vi "ReadSerialised String.vi"(8 "error in (no error)":errorcluster, 11 "object in":refnum<class "Message Class.lvclass">) -> (0 "error out":errorcluster, 2 "Serialised String":string, 3 "object out":refnum<class "Message Class.lvclass">)   [LabVIEW 2018, in "ClientMessaging.lvlib" / "Message Class.lvclass"]
uses:
  Message Class.lvclass
  Message Class.lvclass/Message Class.ctl
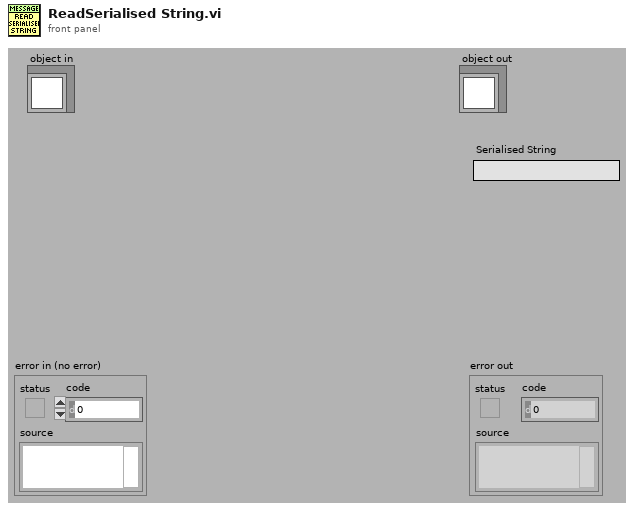
[diagram p1: front panel]
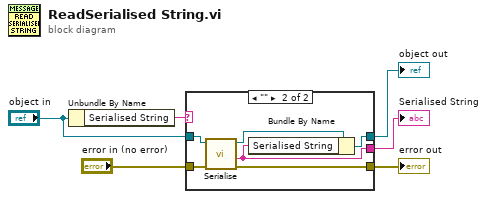
[diagram p0: block diagram]
diagram:
  n1 = Unbundle By Name("object in") -> ("Serialised String"=w6:string)
  n2 = case shown="\"\"" w6 {
    selector: w6 -> [w8 _]
    tunnel: [w9 w12] -> w5
    tunnel: "object in" -> [w9 w15]
    tunnel: "error in (no error)" -> [w7 w13]
    tunnel: [w8 w11] -> w2
    tunnel: [w7 w10] -> w1
    frame "False", Default {
    }
    frame "" {
      n3 = call-dynamic "Serialise.vi"("error in (no error)"=w13, "object in"=w15) -> ("error out"=w10:errorcluster, "Serialised String"=w11:string, "object out"=w14:refnum<class "Message Class.lvclass">)  [unwired: 6 in, 1 out]
      n4 = Bundle By Name(cluster=w14, "Serialised String"=w11) -> (w12:refnum<class "Message Class.lvclass">)
    }
  }
  "error out" <- w1
  "object out" <- w5
  "Serialised String" <- w2
